vi "shutters activate.vi"() -> ()   [LabVIEW 2011]
doc: "Allows manual operation of laser and camera shutters on h-nu microscope"
uses:
  new-h-nu-ixon/Laser type.ctt
  new-h-nu-ixon/Emission filters.ctl
  new-h-nu-ixon/Filter wheel settings globals.vi
  hardware status globals.vi
panel:
  in  "Emission filter wheel":T1
  out "Status":bool
  in  "C off":bool
  in  "C ON":bool
  out "error out":errorcluster
  in  "All Lasers Off":bool
  in  "L0 off 4":bool
  in  "L0 off 3":bool
  in  "L0 off1":bool
  in  "L0 off 0":bool
  in  "L0 ON 4":bool
  in  "L0 ON 3":bool
  in  "L0 ON 2":bool
  in  "Stop":bool
  in  "L0 ON":bool
  out "Lasers Shutters Status":cluster{"Laser":T2, "Status":bool}[](array[cluster])=[{"Laser"=enum."Blue 488 nm", "Status"=FALSE}, {"Laser"=enum."Green 532 nm", "Status"=FALSE}, {"Laser"=enum."Red 633 nm", "Status"=FALSE}, {"Laser"=enum."IR 780", "Status"=FALSE}]
  # "Open"
  # "Close"
  # "Camera"
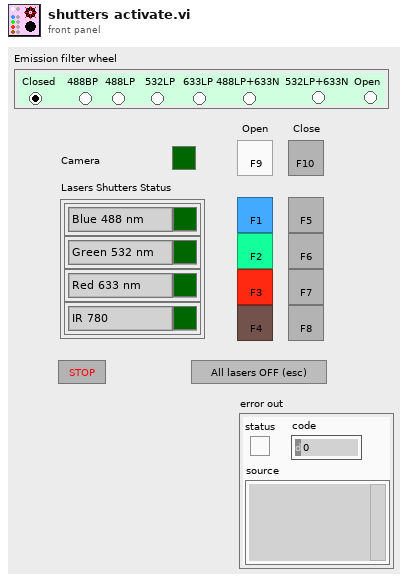
[diagram p1: front panel]
types:
  T1 = typedef "Emission filters.ctl" = enum32{" Closed ", " 488BP ", "488LP", "  532LP ", "633LP", "488LP+633N", "532LP+633N", "Open"}
  T2 = typedef "Laser type.ctt" = enum16{"Blue 488 nm", "Green 532 nm", "Red 633 nm", "IR 780"}
  T3 = typedef "shutters status.ctl" = cluster{"Laser":T2, "Status":bool}[]
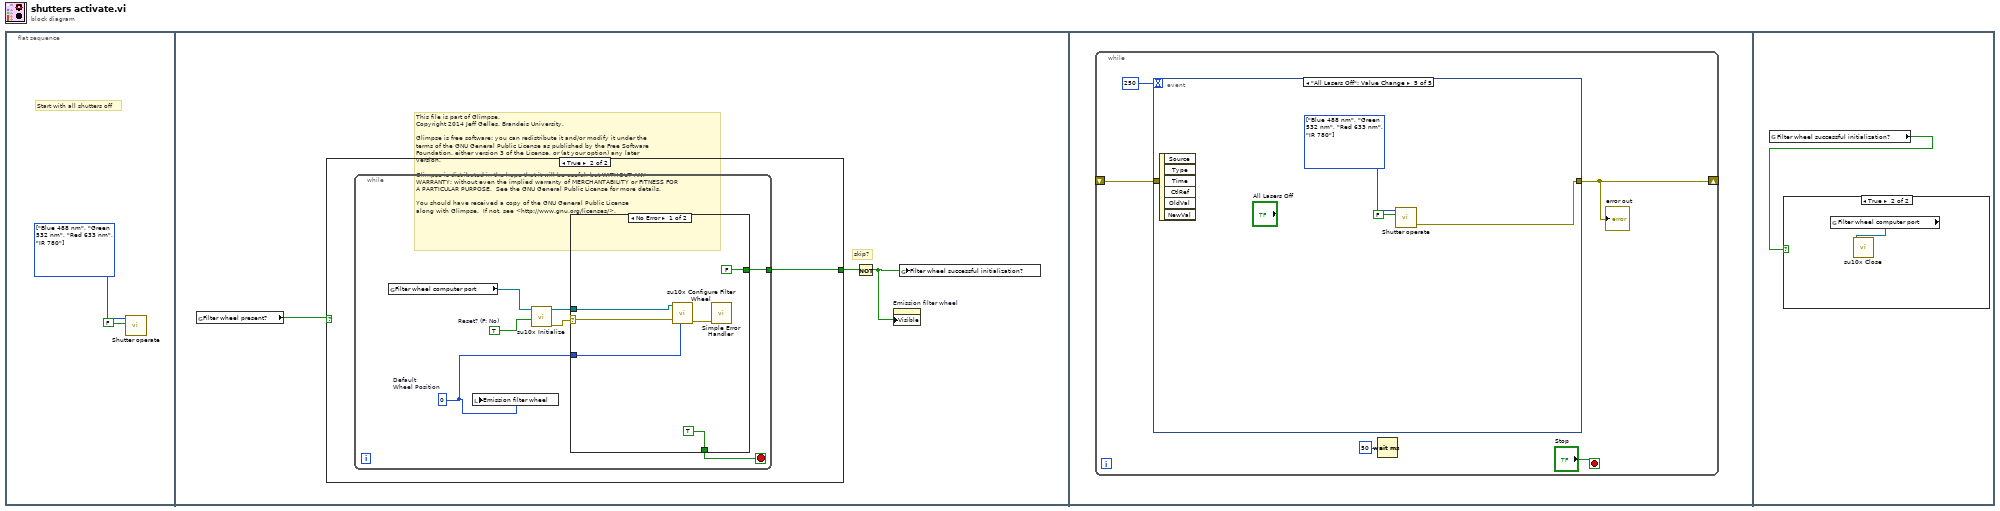
[diagram p0: block diagram]
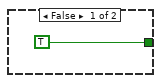
[diagram p2: hidden frame]
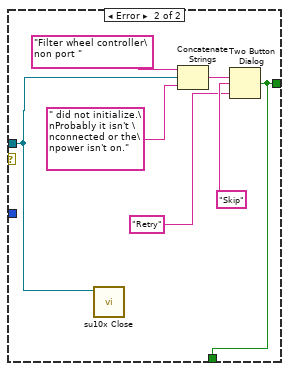
[diagram p3: hidden frame]
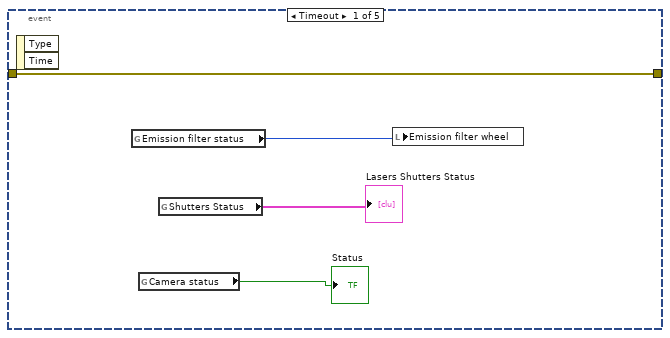
[diagram p4: hidden frame]
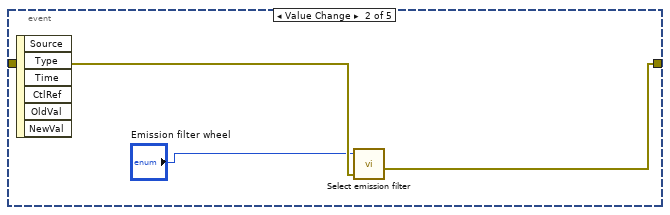
[diagram p5: hidden frame]
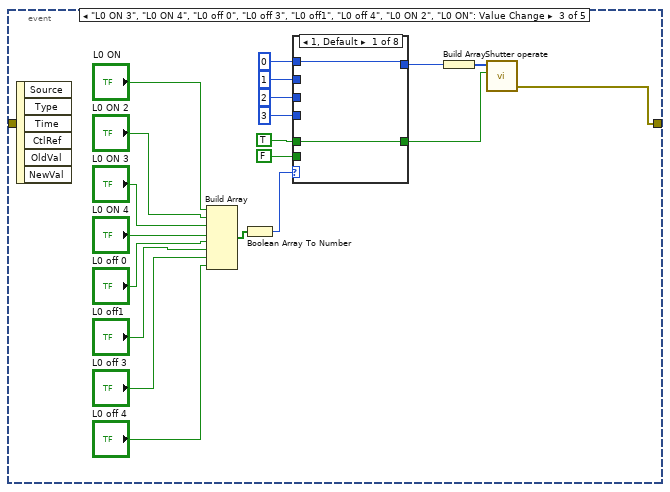
[diagram p6: hidden frame]
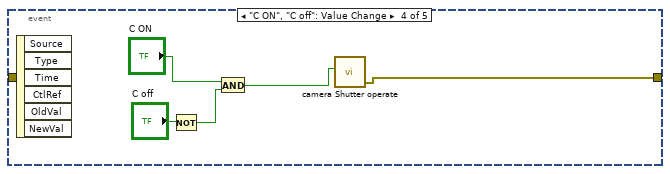
[diagram p14: hidden frame]
diagram:
  # "This file is part of Glimpse. \nCopyright 2014 Jeff Gelles, Brandeis University.    \n\nGlimpse is free software: you can redistribute it and/or modify it under the \nterms of the GNU General Public License as published by the Free Software \nFoundation, either version 3 of the License, or (at your option) any later \nversion.\n\nGlimpse is distributed in the hope that it will be useful, but WITHOUT ANY \nWARRANTY; without even the implied warranty of MERCHANTABILITY or FITNESS FOR \nA PARTICULAR PURPOSE.  See the GNU General Public License for more details.\n\nYou should have received a copy of the GNU General Public License\nalong with Glimpse.  If not, see <http://www.gnu.org/licenses/>."
  n1 = flat-sequence {
    frame #0 {
      w1 = T2[] [enum."Blue 488 nm", enum."Green 532 nm", enum."Red 633 nm", enum."IR 780"] items=["Blue 488 nm", "Green 532 nm", "Red 633 nm", "IR 780"] ("Shutters")
      # "Start with all shutters off"
      n2 = call "Shutter operate.vi"("Shutters"=w1, 2:FALSE) -> ()  [unwired: 1 in, 6 out]
    }
    frame #1 {
      # "skip?"
      n3 = global read "Filter wheel settings globals.vi" "Filter wheel present?"() -> (w3:bool)
      n4 = case shown="True" w3 {
        tunnel: [TRUE ("T button?") w7] -> w4
        frame False {
        }
        frame True {
          n5 = while {
            tunnel: [w9] -> w7
            stop <- w11 stop-if-true
            w8 = u8 0  # Default Wheel Position
            w13 = TRUE  # Reset? (F: No)
            n6 = global read "Filter wheel settings globals.vi" "Filter wheel computer port"() -> (w14:refnum<visa-resource-name>)
            n7 = local write "Emission filter wheel"(w8) -> ()
            n8 = call <instrlib>:"su10x Initialize.vi"("Reset? (F: No)"=w13, "VISA resource name"=w14) -> ("error out"=w12:errorcluster, "VISA resource name out"=w10:refnum<visa-resource-name>)  [unwired: 2 in, 6 out]
            n9 = case shown="No Error" w12 {
              selector: w12 -> [w19 _]
              tunnel: [TRUE w21] -> w11
              tunnel: w10 -> [w18 w22]
              tunnel: [FALSE ("T button?") w21] -> w9
              tunnel: w8 -> [w16 _]
              frame No Error {
                n10 = call <instrlib>:"su10x Configure Filter Wheel.vi"("Wheel Position (0)"=w16, "error in (no error)"=w19, "VISA resource name"=w18) -> ("error out"=w15:errorcluster)  [unwired: 2 in, 6 out]
                n11 = call <vilib>:"Simple Error Handler.vi"("error in (no error)"=w15) -> ()  [unwired: 1 in, 8 out]
              }
              frame Error {
                n12 = call <instrlib>:"su10x Close.vi"("VISA resource name"=w22) -> ()  [unwired: 1 in, 10 out]
                n13 = Concatenate Strings("Filter wheel controller\non port " ("string"), w22, " did not initialize.\nProbably it isn't \nconnected or the\npower isn't on." ("string")) -> (w27:string)
                n14 = Two Button Dialog(message=w27, 1:"Retry" ("F button name (\"Cancel\")"), 2:"Skip" ("T button name (\"OK\")")) -> (T button?=w21:bool)
              }
            }
          }
        }
      }
      n15 = Not(x=w4) -> (.not. x?=w5:bool)
      n16 = property on="Emission filter wheel" class="RadioBtnsControl (strict)"("Visible"=w5) -> ()  [unwired: 2 in, 2 out]
      n17 = global write "Filter wheel settings globals.vi" "Filter wheel successful initialization?"(w5) -> ()
    }
    frame #2 {
      n18 = while {
        shift-right: [w28] -> _
        shift-left: _ -> [w29]
        stop <- "Stop" stop-if-true
        n19 = event shown="[4] \"All Lasers Off\": Value Change" {
          selector: _ -> [_ _ _ _ _]
          dyn-events: _ -> [_ _ _ _ _]
          timeout: 250 -> [_ _ _ _ _]
          tunnel: [w35 w39 w40 w76 w81] -> w28
          tunnel: w29 -> [w35 w38 _ _ _]
          event Timeout {
            n20 = event-data() -> ()  [unwired: 3 out]
            n21 = global read "hardware status globals.vi" "Emission filter status"() -> (w33:T1)
            n22 = global read "hardware status globals.vi" "Camera status"() -> (→"Status":bool)
            n23 = global read "hardware status globals.vi" "Shutters Status"() -> (→"Lasers Shutters Status":T3)
            n24 = local write "Emission filter wheel"(w33) -> ()
          }
          event Value Change {
            n25 = event-data() -> ()  [unwired: 7 out]
            n26 = call "Select emission filter.vi"("Emission filter"="Emission filter wheel", "error in"=w38) -> ("error out"=w39:errorcluster)  [unwired: 4 in]
          }
          event "L0 ON 3", "L0 ON 4", "L0 off 0", "L0 off 3", "L0 off1", "L0 off 4", "L0 ON 2", "L0 ON": Value Change {
            n27 = event-data() -> ()  [unwired: 7 out]
            n28 = Build Array("L0 ON", "L0 ON 2", "L0 ON 3", "L0 ON 4", "L0 off 0", "L0 off1", "L0 off 3", "L0 off 4") -> (w51:bool[])
            n29 = Boolean Array To Number(Boolean array=w51) -> (number=w50:u32)
            n30 = case shown="1, Default" w50 {
              tunnel: [w61 w63 w65 w67 w69 w71 w73 w75] -> w48
              tunnel: 0 -> [w61 _ _ _ w69 _ _ _]
              tunnel: TRUE -> [w60 w62 w64 w66 _ _ _ _]
              tunnel: [w60 w62 w64 w66 w68 w70 w72 w74] -> w45
              tunnel: 1 -> [_ w63 _ _ _ w71 _ _]
              tunnel: 2 -> [_ _ w65 _ _ _ w73 _]
              tunnel: 3 -> [_ _ _ w67 _ _ _ w75]
              tunnel: FALSE -> [_ _ _ _ w68 w70 w72 w74]
              frame 1, Default {
              }
              frame 2 {
              }
              frame 4 {
              }
              frame 8 {
              }
              frame 16 {
              }
              frame 32 {
              }
              frame 64 {
              }
              frame 128 {
              }
            }
            n31 = Build Array(w48) -> (w49:i32[])
            n32 = call "Shutter operate.vi"("Shutters"=w49, 2:w45) -> ("error out"=w40:errorcluster)  [unwired: 1 in, 5 out]
          }
          event "C ON", "C off": Value Change {
            n33 = event-data() -> ()  [unwired: 7 out]
            n34 = Not(x="C off") -> (.not. x?=w79:bool)
            n35 = And(x="C ON", y=w79) -> (x .and. y?=w77:bool)
            n36 = call "camera Shutter operate.vi"("Open?"=w77) -> ("error out"=w76:errorcluster)  [unwired: 1 in, 6 out]
          }
          event "All Lasers Off": Value Change {
            w82 = T2[] [enum."Blue 488 nm", enum."Green 532 nm", enum."Red 633 nm", enum."IR 780"] items=["Blue 488 nm", "Green 532 nm", "Red 633 nm", "IR 780"] ("Shutters")
            n37 = event-data() -> ()  [unwired: 7 out]
            n38 = call "Shutter operate.vi"("Shutters"=w82, 2:FALSE) -> ("error out"=w81:errorcluster)  [unwired: 1 in, 5 out]
          }
        }
        "error out" <- w28
        n39 = Wait (ms)(milliseconds to wait=u32 50) -> ()  [unwired: 1 out]
      }
    }
    frame #3 {
      n40 = global read "Filter wheel settings globals.vi" "Filter wheel successful initialization?"() -> (w84:bool)
      n41 = case shown="True" w84 {
        frame False {
        }
        frame True {
          n42 = global read "Filter wheel settings globals.vi" "Filter wheel computer port"() -> (w85:refnum<visa-resource-name>)
          n43 = call <instrlib>:"su10x Close.vi"("VISA resource name"=w85) -> ()  [unwired: 1 in, 10 out]
        }
      }
    }
  }
